vi "Settings.vi"(8 "Error In":errorcluster, 9 "State In":T2, 10 "Proga Data In":T1={"Station"=[], "Sensor List"=[], "Sensor Id"=[], "Parameters"=["PM10", "PM2.5", "ozon", "dwutlenek azotu", "dwutlenek siarki", "benzen", "tlenek węgla"], "Values"=[110, 75, 180, 200, 350, 21, 15]}, 11 "Main Graph":refnum<vi>) -> (0 "Error Out":errorcluster, 1 "State Out":T2, 2 "Prog Data Out":T1={"Station"=[], "Sensor List"=[], "Sensor Id"=[], "Parameters"=["PM10", "PM2.5", "ozon", "dwutlenek azotu", "dwutlenek siarki", "benzen", "tlenek węgla"], "Values"=[110, 75, 180, 200, 350, 21, 15]})   [LabVIEW 2020]
doc: "This VI allows change colors on main xy graph, add visible standards for specific parameters and reload station."
uses:
  Ctrls/ProgData.ctl
  Ctrls/StateMachineEnum.ctl
  user32.dll
panel:
  in  "Close":bool
  out "TitleBar":bool
  in  "Slide":u32(slide) scale=0.0..6.0
  in  "Values":i32[](array[numeric])=[110, 75, 180, 200, 350, 21, 15] caption="Wartość:"
  in  "Parameters":string[](array[string])=["PM10", "PM2.5", "ozon", "dwutlenek azotu", "dwutlenek siarki", "benzen", "tlenek węgla"] caption="Parametr:"
  in  "Select":bool
  in  "Standard_V":bool=TRUE
  in  "Standards_C":u32(colorbox)=16711680 caption="Kolor lini progu"
  in  "Point_C":u32(colorbox)=16777224 caption="Kolor punktów na wykresie"
  in  "Plot_C":u32(colorbox)=16777224 caption="Kolor lini wykresu"
  # "Progi dla parametrów"
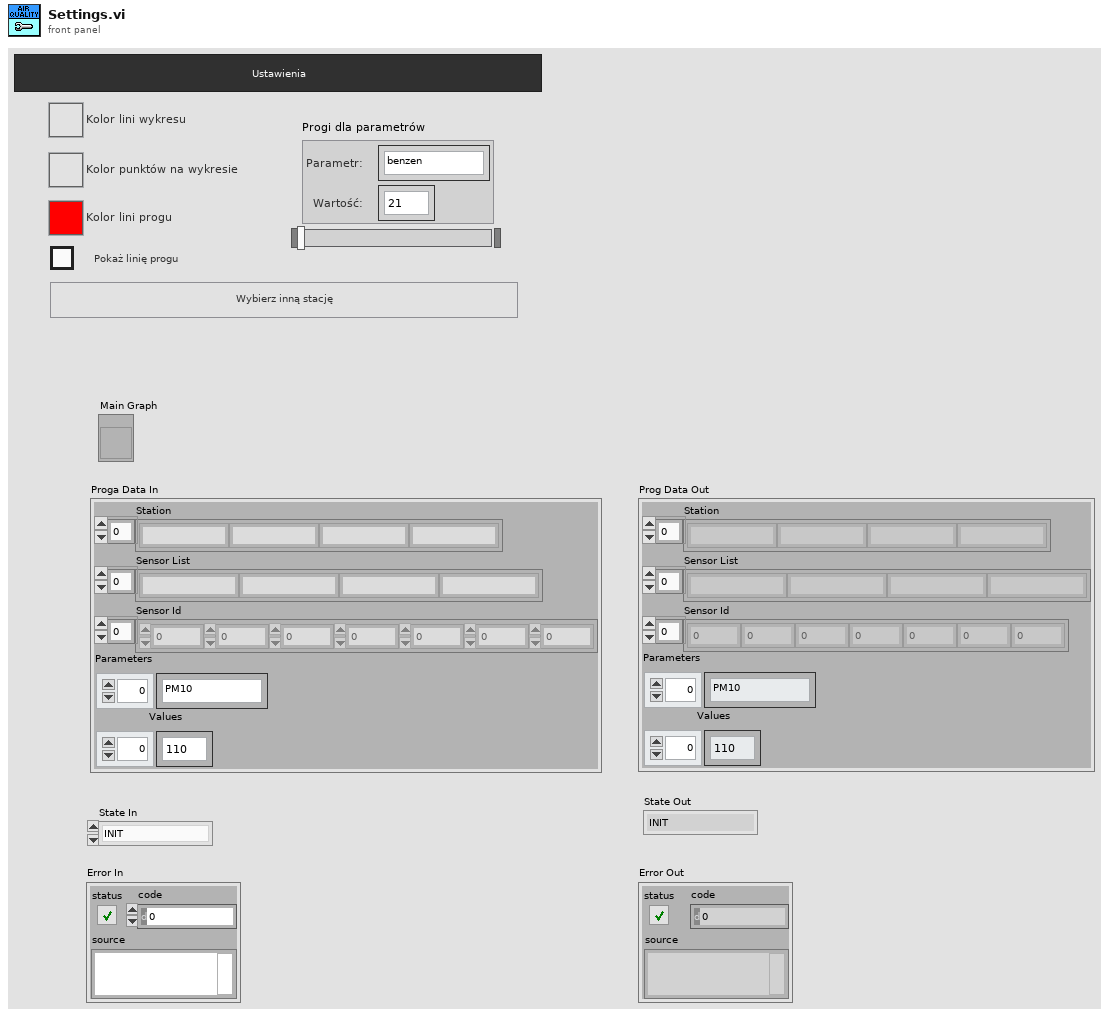
[diagram p1: front panel]
types:
  T1 = typedef "ProgData.ctl" = cluster{"Station":string[], "Sensor List":string[], "Sensor Id":dbl[], "Parameters":string[], "Values":i32[]}
  T2 = typedef "StateMachineEnum.ctl" = enum16{"INIT", "IDLE", "GET DATA", "ERROR HANDLER", "CLOSE"}
  T3 = enum32{"Invalid", "Standard", "Closed", "Hidden", "Minimized", "Maximized"}
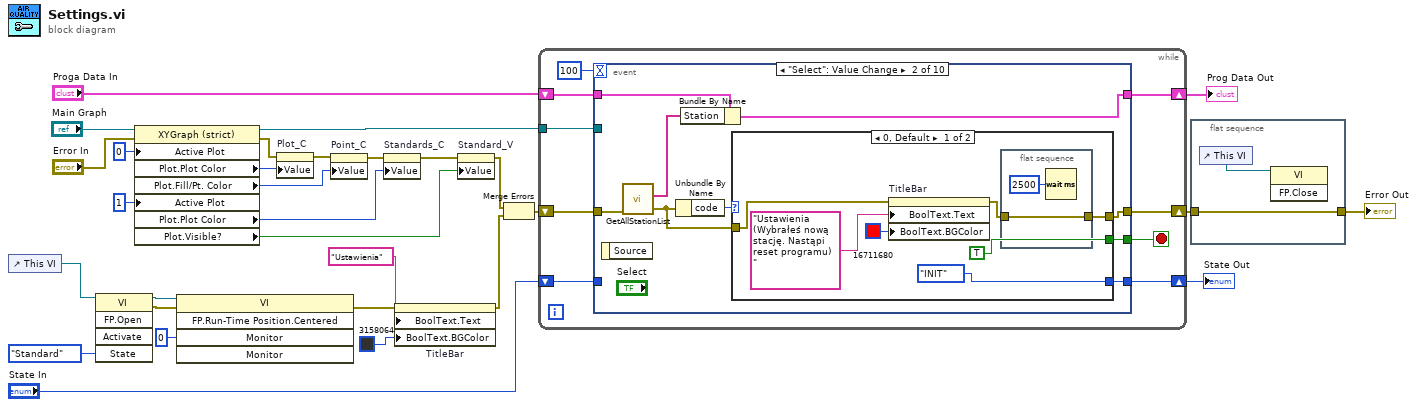
[diagram p0: block diagram]
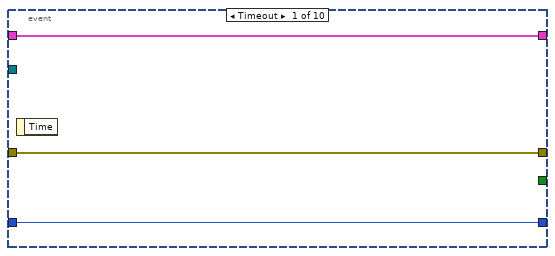
[diagram p2: hidden frame]
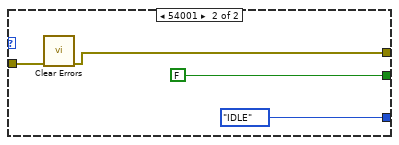
[diagram p3: hidden frame]
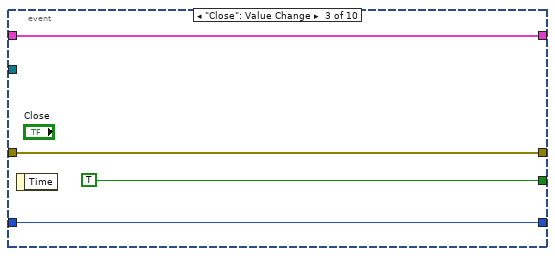
[diagram p4: hidden frame]
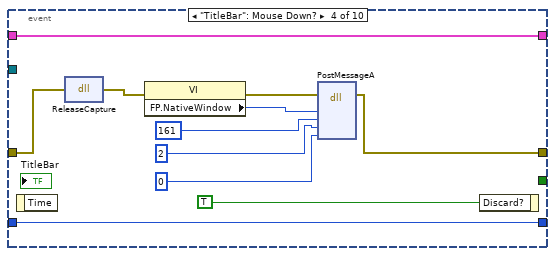
[diagram p5: hidden frame]
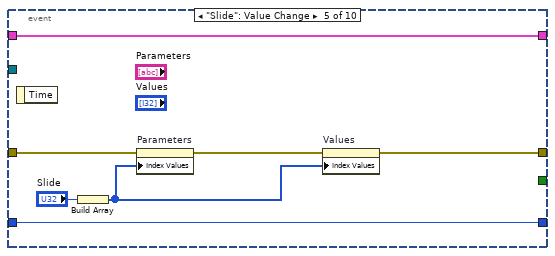
[diagram p6: hidden frame]
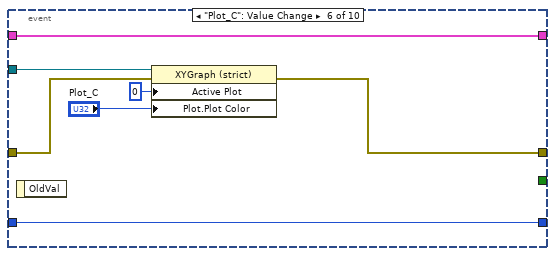
[diagram p7: hidden frame]
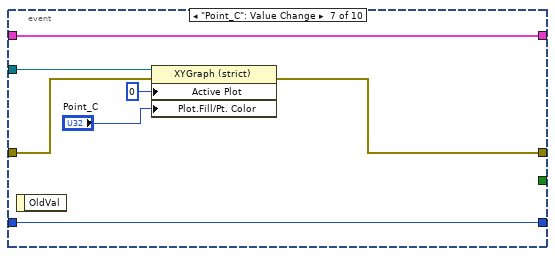
[diagram p8: hidden frame]
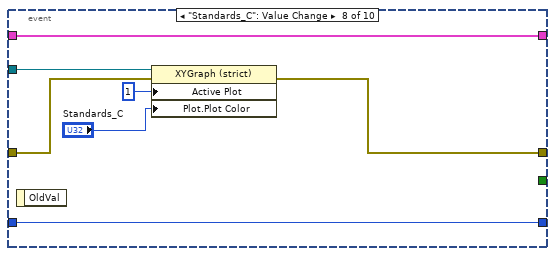
[diagram p9: hidden frame]
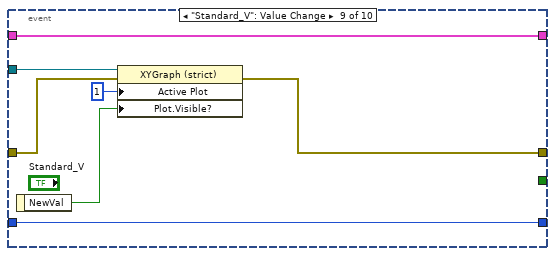
[diagram p10: hidden frame]
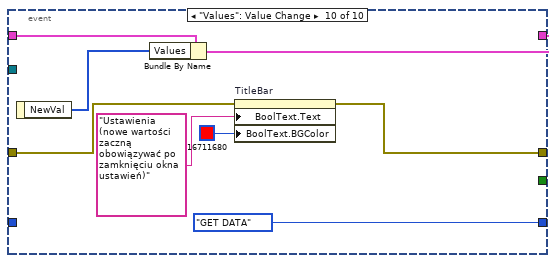
[diagram p11: hidden frame]
diagram:
  n1 = control-ref of="This VI"() -> (w30:refnum<vi>)
  n2 = invoke class="VI" method="FP.Open"(reference=w30, "State"=T3."Standard") -> (reference out=w2:refnum<vi>, error out=w9:errorcluster)  [unwired: 3 in, 3 out]
  n3 = property class="XYGraph (strict)"(reference="Main Graph", error in="Error In", "Active Plot"=u32 0, "Active Plot"=u32 1) -> (reference out=w23:refnum<vi>, error out=w22:errorcluster, "Plot.Plot Color"=w20:u32, "Plot.Fill/Pt. Color"=w19:u32, "Plot.Plot Color"=w16:u32, "Plot.Visible?"=w15:bool)
  n4 = invoke class="VI" method="FP.Run-Time Position.Centered"(reference=w2, error in=w9, "Monitor"=i16 0) -> (error out=w3:errorcluster)  [unwired: 2 in, 4 out]
  n5 = property on="Plot_C" class="ColBox"(error in=w22, "Value"=w20) -> (error out=w21:errorcluster)  [unwired: 1 in, 1 out]
  n6 = property on="Point_C" class="ColBox"(error in=w21, "Value"=w19) -> (error out=w17:errorcluster)  [unwired: 1 in, 1 out]
  n7 = property on="Standards_C" class="ColBox"(error in=w17, "Value"=w16) -> (error out=w14:errorcluster)  [unwired: 1 in, 1 out]
  n8 = property on="TitleBar" class="Bool (strict)"(error in=w3, "BoolText.Text"="Ustawienia" ("Boolean Text.Text"), "BoolText.BGColor"=u32 3158064 ("Boolean Text.Text Colors:BG Color")) -> (error out=w8:errorcluster)  [unwired: 1 in, 1 out]
  n9 = property on="Standard_V" class="Bool (strict)"(error in=w14, "Value"=w15) -> (error out=w12:errorcluster)  [unwired: 1 in, 1 out]
  n10 = Merge Errors(w12, w8) -> (w13:errorcluster)
  n11 = while {
    shift-right: [w35] -> w5
    shift-left: w13 -> [w38]
    tunnel: w23 -> [w37]
    shift-right: [w33] -> w10
    shift-left: "State In" -> [w34]
    shift-right: [w31] -> w26
    shift-left: "Proga Data In" -> [w32]
    stop <- w36 stop-if-true
    n12 = event shown="[1] \"Select\": Value Change" {
      selector: _ -> [_ _ _ _ _ _ _ _ _ _]
      dyn-events: _ -> [_ _ _ _ _ _ _ _ _ _]
      timeout: 100 -> [_ _ _ _ _ _ _ _ _ _]
      tunnel: w38 -> [w42 w51 w67 w71 w86 w90 w98 w105 w112 w117]
      tunnel: w37 -> [_ _ _ _ _ w93 w100 w107 w113 _]
      tunnel: [_ w45 TRUE _ _ _ _ _ _ _] -> w36
      tunnel: [w42 w43 w67 w70 w84 w89 w97 w104 w111 w116] -> w35
      tunnel: w34 -> [w40 _ w68 w79 w80 w88 w96 w103 w109 _]
      tunnel: [w40 w44 w68 w79 w80 w88 w96 w103 w109 StateMachineEnum."GET DATA" ("State In")] -> w33
      tunnel: w32 -> [w41 w50 w66 w69 w81 w87 w94 w101 w108 w121]
      tunnel: [w41 w49 w66 w69 w81 w87 w94 w101 w108 w119] -> w31
      event Timeout {
        n13 = event-data() -> ()  [unwired: 1 in, 1 out]
      }
      event "Select": Value Change {
        n14 = event-data() -> ()  [unwired: 1 in, 1 out]
        n15 = call "GetAllStationList.vi"("Error In"=w51) -> ("Error Out"=w46:errorcluster, "Station"=w48:string[])  [unwired: 9 in]
        n16 = Unbundle By Name(w46) -> ("code"=w47:i32)
        n17 = Bundle By Name(cluster=w50, "Station"=w48) -> (w49:T1)
        n18 = case shown="0, Default" w47 {
          tunnel: w46 -> [w58 w64]
          tunnel: [TRUE FALSE] -> w45
          tunnel: [StateMachineEnum."INIT" ("State In") StateMachineEnum."IDLE" ("State In")] -> w44
          tunnel: [w52 w61] -> w43
          frame 0, Default {
            n19 = property on="TitleBar" class="Bool (strict)"(error in=w58, "BoolText.Text"="Ustawienia (Wybrałeś nową stację. Nastąpi reset programu) " ("Boolean Text.Text"), "BoolText.BGColor"=u32 16711680 ("Boolean Text.Text Colors:BG Color")) -> (error out=w53:errorcluster)  [unwired: 1 in, 1 out]
            n20 = flat-sequence {
              tunnel: w53 -> [w59]
              tunnel: [w59] -> w52
              frame #0 {
                n21 = Wait (ms)(milliseconds to wait=u32 2500) -> ()  [unwired: 1 out]
              }
            }
          }
          frame 54001 {
            n22 = call <vilib>:"Clear Errors.vi"("error in (no error)"=w64) -> ("error out"=w61:errorcluster)  [unwired: 5 in, 1 out]
          }
        }
      }
      event "Close": Value Change {
        n23 = event-data() -> ()  [unwired: 1 in, 1 out]
      }
      event "TitleBar": Mouse Down? {
        n24 = event-data() -> ()  [unwired: 1 in, 1 out]
        n25 = dll-call lib="user32.dll" fn="ReleaseCapture"(error in=w71) -> (error out=w75:errorcluster)  [unwired: 3 in, 1 out]
        n26 = property class="VI"(error in=w75) -> (error out=w76:errorcluster, "FP.NativeWindow"=w77:u64)  [unwired: 1 in, 1 out]
        n27 = dll-call lib="user32.dll" fn="PostMessageA"(error in=w76, "hWnd"=w77, "Msg"=161, "wParam"=2, "lParam"=0) -> (error out=w70:errorcluster)  [unwired: 7 in, 1 out]
        n28 = event-data("Discard?"=TRUE) -> ()  [unwired: 1 in, 1 out]
      }
      event "Slide": Value Change {
        n29 = event-data() -> ()  [unwired: 1 in, 1 out]
        n30 = Build Array("Slide") -> (w82:u32[])
        n31 = property on="Parameters" class="Arr (strict)"(error in=w86, "Index Values"=w82) -> (error out=w85:errorcluster)  [unwired: 1 in, 1 out]
        n32 = property on="Values" class="Arr (strict)"(error in=w85, "Index Values"=w82) -> (error out=w84:errorcluster)  [unwired: 1 in, 1 out]
      }
      event "Plot_C": Value Change {
        n33 = event-data() -> ()  [unwired: 1 in, 1 out]
        n34 = property class="XYGraph (strict)"(reference=w93, error in=w90, "Active Plot"=u32 0, "Plot.Plot Color"="Plot_C") -> (error out=w89:errorcluster)  [unwired: 1 out]
      }
      event "Point_C": Value Change {
        n35 = event-data() -> ()  [unwired: 1 in, 1 out]
        n36 = property class="XYGraph (strict)"(reference=w100, error in=w98, "Active Plot"=u32 0, "Plot.Fill/Pt. Color"="Point_C") -> (error out=w97:errorcluster)  [unwired: 1 out]
      }
      event "Standards_C": Value Change {
        n37 = event-data() -> ()  [unwired: 1 in, 1 out]
        n38 = property class="XYGraph (strict)"(reference=w107, error in=w105, "Active Plot"=u32 1, "Plot.Plot Color"="Standards_C") -> (error out=w104:errorcluster)  [unwired: 1 out]
      }
      event "Standard_V": Value Change {
        n39 = event-data() -> ("NewVal"=w110:bool)  [unwired: 1 in]
        n40 = property class="XYGraph (strict)"(reference=w113, error in=w112, "Active Plot"=u32 1, "Plot.Visible?"=w110) -> (error out=w111:errorcluster)  [unwired: 1 out]
      }
      event "Values": Value Change {
        n41 = event-data() -> ("NewVal"=w120:i32[])  [unwired: 1 in]
        n42 = Bundle By Name(cluster=w121, "Values"=w120) -> (w119:T1)
        n43 = property on="TitleBar" class="Bool (strict)"(error in=w117, "BoolText.Text"="Ustawienia (nowe wartości zaczną obowiązywać po zamknięciu okna ustawień)" ("Boolean Text.Text"), "BoolText.BGColor"=u32 16711680 ("Boolean Text.Text Colors:BG Color")) -> (error out=w116:errorcluster)  [unwired: 1 in, 1 out]
      }
    }
  }
  "Prog Data Out" <- w26
  "State Out" <- w10
  n44 = flat-sequence {
    tunnel: w5 -> [w123]
    tunnel: [w123] -> w4
    frame #0 {
      n45 = control-ref of="This VI"() -> (w124:refnum<vi>)
      n46 = invoke class="VI" method="FP.Close"(reference=w124) -> ()  [unwired: 2 in, 3 out]
    }
  }
  "Error Out" <- w4
